vi "UGID.vi"(8 "error in (no error)":errorcluster, 11 "IncludeDatatime":bool) -> (0 "error out":errorcluster, 2 "error":i32, 3 "result string":string)   [LabVIEW 2021]
uses:
  <resource>/Framework/Providers/mxLvProvider.mxx
panel:
  out "length":i32
  out "value":string
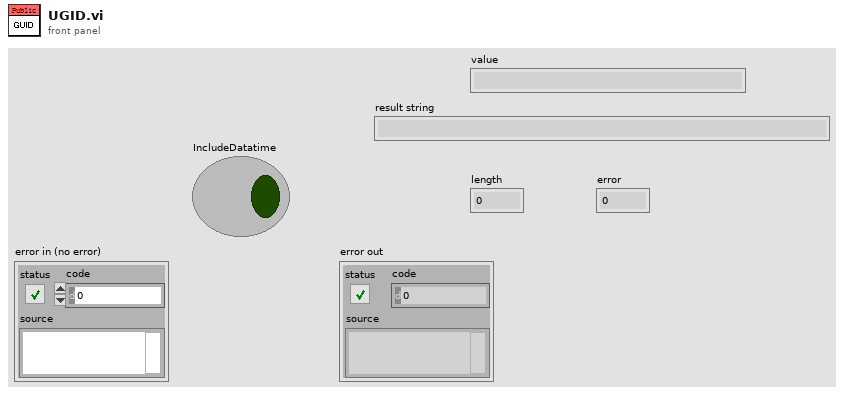
[diagram p1: front panel]
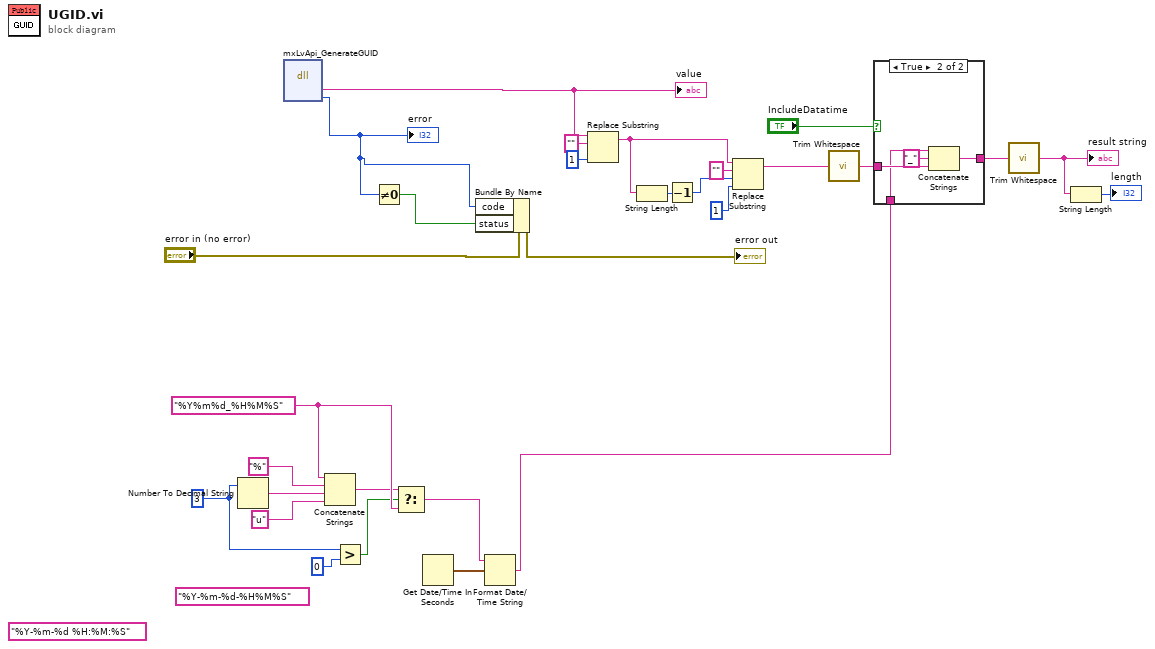
[diagram p0: block diagram]
diagram:
  w10 = 3 ("u?")
  (unwired) "%Y-%m-%d %H:%M:%S" ("time format string (%c)")
  (unwired) "%Y-%m-%d-%H%M%S" ("time format string (%c)")
  w14 = "%Y%m%d_%H%M%S" ("time format string (%c)")
  n1 = Number To Decimal String(number=w10) -> (decimal integer string=w9:string)  [unwired: 1 in]
  n2 = dll-call lib="C:/Program Files (x86)/National Instruments/LabVIEW 2021/resource/Framework/Providers/mxLvProvider.mxx" fn="mxLvApi_GenerateGUID"() -> ("value"=w29:string, "error"=w16:i32)  [unwired: 3 in, 5 out]
  "value" <- w29
  "error" <- w16
  n3 = Concatenate Strings(w14, "%" ("string"), w9, "u" ("string")) -> (w13:string)
  n4 = Greater?(x=w10, y=0) -> (0:w12:bool)
  n5 = Not Equal To 0?(x=w16) -> (x != 0?=w17:bool)
  n6 = Select(t=w13, s=w12, f=w14) -> (s? t:f=w6:string)
  n7 = Get Date/Time In Seconds() -> (seconds since 1Jan1904=w15:timestamp)
  n8 = Bundle By Name(cluster="error in (no error)", "code"=w16, "status"=w17) -> (→"error out":errorcluster)
  n9 = Format Date/Time String(time format string (%c)=w6, seconds (now)=w15) -> (date/time string=w4:string)  [unwired: 1 in]
  n10 = Replace Substring(2:1 ("length (len. of substring)"), 4:"" ("substring (\"\")"), 5:w29) -> (1:w22:string)  [unwired: 1 in, 1 out]
  n11 = String Length(string=w22) -> (length=w24:i32)
  n12 = Decrement(x=w24) -> (x-1=w23:i32)
  n13 = Replace Substring(2:1 ("length (len. of substring)"), 3:w23, 4:"" ("substring (\"\")"), 5:w22) -> (1:w21:string)  [unwired: 1 out]
  n14 = call <vilib>:"Trim Whitespace.vi"("string"=w21) -> ("trimmed string"=w20:string)  [unwired: 1 in]
  n15 = case shown="True" "IncludeDatatime" {
    tunnel: w20 -> [w30 w34]
    tunnel: [w30 w33] -> w5
    tunnel: w4 -> [_ w32]
    frame False {
    }
    frame True {
      n16 = Concatenate Strings(w32, "_" ("string"), w34) -> (w33:string)
    }
  }
  n17 = call <vilib>:"Trim Whitespace.vi"("string"=w5) -> ("trimmed string"=w2:string)  [unwired: 1 in]
  "result string" <- w2
  n18 = String Length(string=w2) -> (length=→"length":i32)
